vi "K-C (SubVI).vi"(11 "Град F":dbl) -> (3 "Град C":dbl)   [LabVIEW 2020]
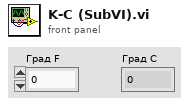
[diagram p1: front panel]
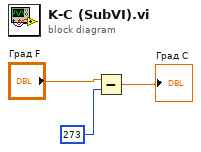
[diagram p0: block diagram]
diagram:
  n1 = Subtract(x="Град F", y=273) -> (x-y=→"Град C":dbl)
